vi "Pre-Build VI - Run Unit Tests.vi"(8 "error in (no error)":errorcluster) -> (0 "error out":errorcluster, 1 "VIs without test coverage":string[](array[string]), 2 "error type":enum16{"fatal", "non-fatal", "warning"}(ring))   [LabVIEW 2009]
uses:
  <userlib>/_OpenG.lib/array/array.llb/Empty 1D Array (String)__ogtk.vi
  <userlib>/_OpenG.lib/array/array.llb/Filter 1D Array (String)__ogtk.vi
  <userlib>/_OpenG.lib/file/file.llb/Build Path - Traditional__ogtk.vi
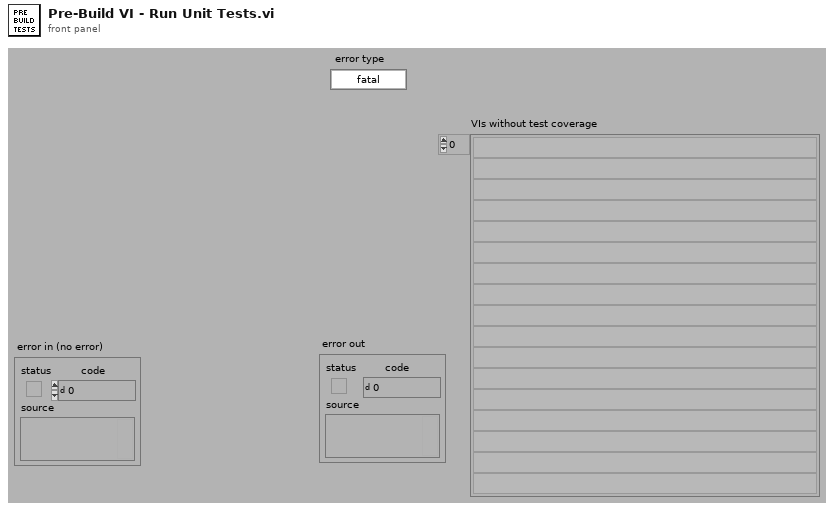
[diagram p1: front panel]
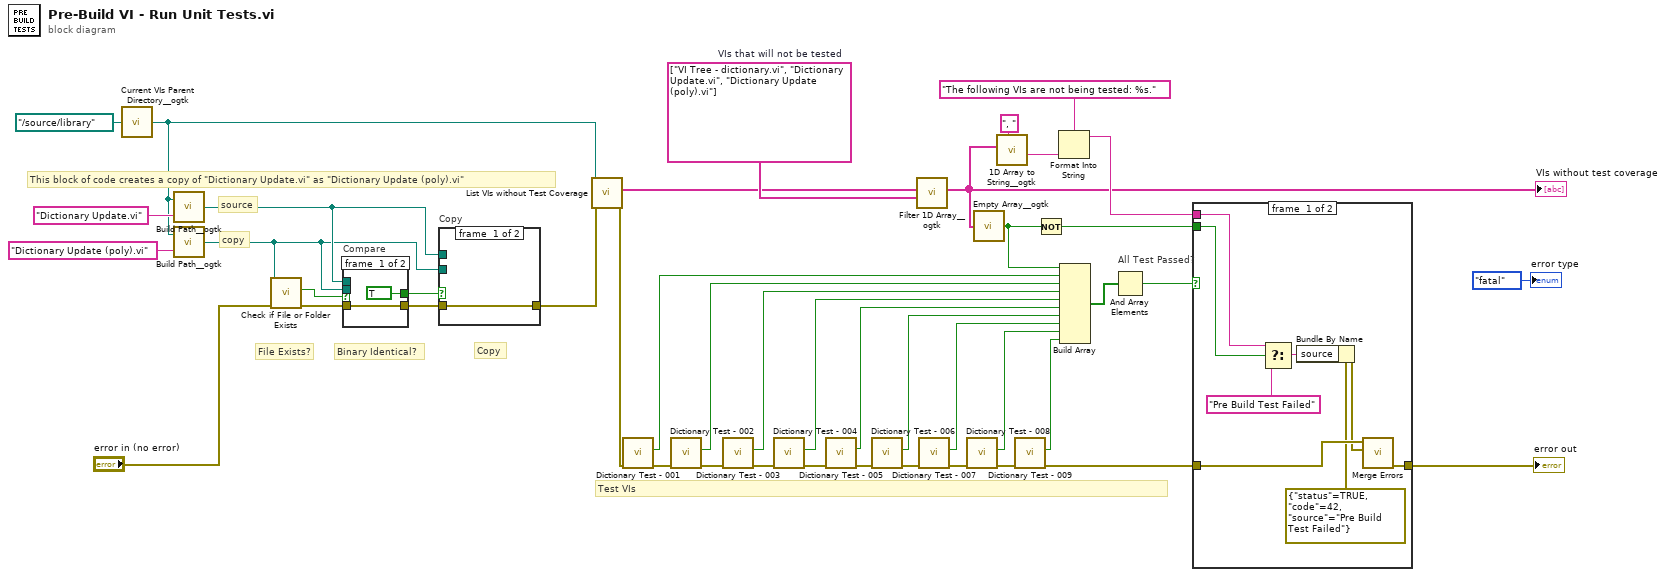
[diagram p0: block diagram]
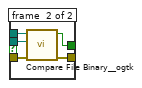
[diagram p2: hidden frame]
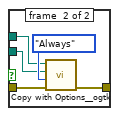
[diagram p3: hidden frame]
diagram:
  w36 = string[] ["VI Tree - dictionary.vi", "Dictionary Update.vi", "Dictionary Update (poly).vi"]  # VIs that will not be tested
  # "This block of code creates a copy of \"Dictionary Update.vi\" as \"Dictionary Update (poly).vi\""
  # "copy"
  # "source"
  # "Copy"
  # "Binary Identical?"
  # "File Exists?"
  # "All Test Passed?"
  # "Test VIs"
  n1 = call <userlib>:"Current VIs Parent Directory__ogtk.vi"("Relative path (.)"=path "../source/library") -> ("Parent Directory (+ Relative)"=w8:path)  [unwired: 4 in]
  n2 = call-poly <userlib>:"Build Path__ogtk.vi"("name or relative path"="Dictionary Update.vi", "base path"=w8) -> ("appended path"=w7:path)
  n3 = call-poly <userlib>:"Build Path__ogtk.vi"("name or relative path"="Dictionary Update (poly).vi", "base path"=w8) -> ("appended path"=w2:path)
  n4 = call <vilib>:"Check if File or Folder Exists.vi"("error in (no error)"="error in (no error)", "path"=w2) -> ("error out"=w3:errorcluster, "file or folder exists?"=w1:bool)  [unwired: 7 in, 1 out]
  n5 = case "Compare" shown="True" w1 {
    tunnel: w7 -> [_ w51]
    tunnel: [w45 w50] -> w6
    tunnel: [TRUE ("not equal") w49] -> w5
    tunnel: w3 -> [w45 w48]
    tunnel: w2 -> [_ w47]
    frame #0 {
    }
    frame #1 {
      n6 = call <userlib>:"Compare File Binary__ogtk.vi"("error in (no error)"=w48, "copy file"=w47, "original file"=w51) -> ("error out"=w50:errorcluster, "not equal"=w49:bool)  [unwired: 3 in]
    }
  }
  n7 = case "Copy" shown="False" w5 {
    tunnel: [w52 w57] -> w11
    tunnel: w7 -> [_ w55]
    tunnel: w2 -> [_ w54]
    tunnel: w6 -> [w52 w53]
    frame #0 {
    }
    frame #1 {
      n8 = call <userlib>:"Copy with Options__ogtk.vi"("error in (no error)"=w53, "Replace Mode (Never)"=enum16{"Never", "Always", "If Newer"}."Always", "target path"=w54, "source path"=w55) -> ("error out"=w57:errorcluster)  [unwired: 6 in, 1 out]
    }
  }
  n9 = call "List VIs without Test Coverage.vi"("error in (no error)"=w11, "Source Root"=w8) -> ("error out"=w37:errorcluster, "VIs without test coverage"=w35:string[])  [unwired: 8 in]
  n10 = call "Dictionary Test - 001.vi"("error in (no error)"=w37) -> ("error out"=w39:errorcluster, "pass"=w43:bool)  [unwired: 9 in]
  n11 = call "Dictionary Test - 002.vi"("error in (no error)"=w39) -> ("error out"=w28:errorcluster, "pass"=w38:bool)  [unwired: 9 in]
  n12 = call "Dictionary Test - 003.vi"("error in (no error)"=w28) -> ("error out"=w26:errorcluster, "pass"=w27:bool)  [unwired: 9 in]
  n13 = call "Dictionary Test - 004.vi"("error in (no error)"=w26) -> ("error out"=w23:errorcluster, "pass"=w25:bool)  [unwired: 9 in]
  n14 = call "Dictionary Test - 005.vi"("error in (no error)"=w23) -> ("error out"=w22:errorcluster, "pass"=w20:bool)  [unwired: 9 in]
  n15 = call "Dictionary Test - 006.vi"("error in (no error)"=w22) -> ("error out"=w21:errorcluster, "pass"=w19:bool)  [unwired: 9 in]
  n16 = call-poly <userlib>:"Filter 1D Array__ogtk.vi"("Items to Filter"=w36, "String Array"=w35) -> ("Filtered String Array"=w12:string[])  [unwired: 5 in]
  "VIs without test coverage" <- w12
  n17 = call "Dictionary Test - 007.vi"("error in (no error)"=w21) -> ("error out"=w17:errorcluster, "pass"=w18:bool)  [unwired: 9 in]
  n18 = call "Dictionary Test - 008.vi"("error in (no error)"=w17) -> ("error out"=w16:errorcluster, "pass"=w14:bool)  [unwired: 9 in]
  n19 = call-poly <userlib>:"Empty Array__ogtk.vi"("Array"=w12) -> ("Empty Array?"=w30:bool)  [unwired: 8 in]
  n20 = call <userlib>:"1D Array to String__ogtk.vi"("delimiter (Tab)"=", ", "Array of Strings"=w12) -> ("delimited string"=w33:string)  [unwired: 9 in]
  n21 = call "Dictionary Test - 009.vi"("error in (no error)"=w16) -> ("error out"=w15:errorcluster, "pass"=w13:bool)  [unwired: 9 in]
  n22 = Not(x=w30) -> (.not. x?=w29:bool)
  n23 = Format Into String(format string="The following VIs are not being tested: %s.", w33) -> (resulting string=w31:string)  [unwired: 2 in, 1 out]
  n24 = Build Array(w30, w43, w38, w27, w25, w20, w19, w18, w14, w13) -> (w42:bool[])
  n25 = And Array Elements(Boolean array=w42) -> (logical AND=w41:bool)
  n26 = case shown="False" w41 {
    tunnel: w15 -> [w65 w66]
    tunnel: [w64 w66] -> w40
    tunnel: w29 -> [w63 _]
    tunnel: w31 -> [w62 _]
    frame #0 {
      n27 = Select(t=w62, s=w63, f="Pre Build Test Failed" ("source")) -> (s? t:f=w60:string)
      n28 = Bundle By Name(cluster=errorcluster {"status"=TRUE, "code"=42, "source"="Pre Build Test Failed"} ("error out"), "source"=w60) -> (w59:errorcluster)
      n29 = call <vilib>:"Merge Errors.vi"("error in 2 (no error)"=w59, "error in 1 (no error)"=w65) -> ("error out"=w64:errorcluster)  [unwired: 5 in]
    }
    frame #1 {
    }
  }
  "error out" <- w40
  "error type" <- enum16{"fatal", "non-fatal", "warning"}."fatal" ("error type")
